vi "File - calendar tree.vi"(8 "error in (no error)":errorcluster) -> (0 "error out":errorcluster)   [LabVIEW 2026, in "Tests.lvlib"]
doc: "Integration test (Caraya). Verifies a statement logged through the Logger reaches a single registered appender. Launches a manager with the default file disabled and a queue-mode relay capture probe (Open Test Mgr), logs one INFO statement, dequeues from the capture queue with a timeout, and asserts it was delivered and its message matches. Tears down with Close Test Mgr regardless of assertion outcome (SRS-LMBR-019). Uses the manager fixture; no temp root needed.\n\nImplements LMBR-T-029 -> SRS-019. Assert-level IDs: Test-ID-Assert-Checklist.md."
uses:
  Tests.lvlib
  src/TypeDefs/Severity.ctl
  src/TypeDefs/FileAppenderConfig.ctl
  src/TypeDefs/AppenderConfig.ctl
  src/TypeDefs/Filter.ctl
  src/TypeDefs/FilterMode.ctl
  src/TypeDefs/DropPolicy.ctl
  src/TypeDefs/FileConfig.ctl
  <vilib>/addons/_JKI Toolkits/Caraya/classes/Assert/Assert False.vi
  <vilib>/addons/_JKI Toolkits/Caraya/classes/Assert/Assert True.vi
  <vilib>/addons/_JKI Toolkits/Caraya/classes/Test/Test.lvclass
  src/Lumberjack.lvlib
  src/Public/Logger.lvclass/Logger.lvclass
  <vilib>/addons/_JKI Toolkits/Caraya/classes/Assert/Assert.lvclass
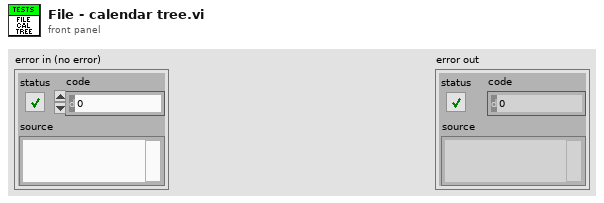
[diagram p1: front panel]
types:
  T1 = typedef "Lumberjack.lvlib/Severity.ctl" = enum16{"OFF", "FATAL", "ERROR", "WARN", "INFO", "DEBUG", "TRACE", "ALL"}
  T2 = typedef "Lumberjack.lvlib/FileAppenderConfig.ctl" = cluster{"common":T3, "file":T7}
  T3 = typedef "Lumberjack.lvlib/AppenderConfig.ctl" = cluster{"id":string, "threshold":T1, "filter":T4, "queueBound":i32, "dropPolicy":T6, "useUTC":bool}
  T4 = typedef "Lumberjack.lvlib/Filter.ctl" = cluster{"mode":T5, "levelMin":T1, "levelMax":T1, "tagPrefix":string}
  T5 = typedef "Lumberjack.lvlib/FilterMode.ctl" = enum16{"Mirror", "Routed"}
  T6 = typedef "Lumberjack.lvlib/DropPolicy.ctl" = enum16{"DropOldest", "DropNewest", "LevelAware"}
  T7 = typedef "Lumberjack.lvlib/FileConfig.ctl" = cluster{"rootFolder":path, "maxFileSize":i64, "maxFileCount":i32, "baseName":string, "extension":string, "delimiter":string, "calendarFolderTree":bool}
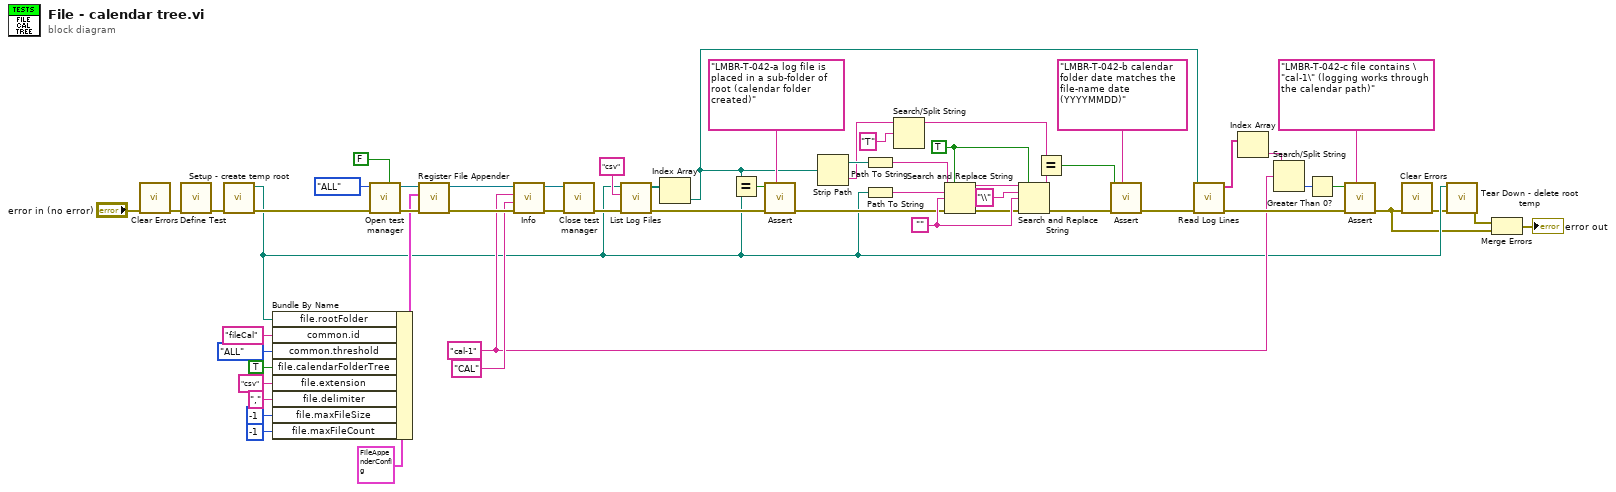
[diagram p0: block diagram]
diagram:
  w19 = TRUE ("replace all? (F)")
  w21 = ""
  w30 = "cal-1" ("message")
  n1 = call <vilib>:"Clear Errors.vi"("error in (no error)"="error in (no error)") -> ("error out"=w5:errorcluster)  [unwired: 5 in, 1 out]
  n2 = call <vilib>:"Define Test.vi"("error in (no error)"=w5) -> ("error out"=w57:errorcluster)  [unwired: 9 in, 1 out]
  n3 = call "Setup - create temp root.vi"("error in (no error)"=w57) -> ("error out"=w27:errorcluster, "tempRoot"=w8:path)  [unwired: 9 in]
  n4 = Bundle By Name(cluster=T2 {"common"={"id"="", "threshold"=enum."INFO", "filter"={"mode"=enum."Mirror", "levelMin"=enum."INFO", "levelMax"=enum."INFO", "tagPrefix"=""}, "queueBound"=0, "dropPolicy"=enum."DropOldest", "useUTC"=FALSE}, "file"={"rootFolder"=path "", "maxFileSize"=0, "maxFileCount"=0, "baseName"="", "extension"="", "delimiter"="", "calendarFolderTree"=FALSE}} ("FileAppenderConfig"), "file.rootFolder"=w8, "common.id"="fileCal", "common.threshold"=Severity."ALL", "file.calendarFolderTree"=TRUE, "file.extension"="csv", "file.delimiter"=",", "file.maxFileSize"=i64 -1, "file.maxFileCount"=-1) -> (w51:T2)
  n5 = call "Open test manager.vi"("enableDefaultFile"=FALSE, "error in (no error)"=w27, "globalThreshold"=Severity."ALL") -> ("error out"=w55:errorcluster, "Logger out"=w50:refnum<class "Logger.lvclass">)  [unwired: 7 in]
  n6 = call "Register File Appender.vi"("error in (no error)"=w55, "FileAppenderConfig"=w51, "Logger in"=w50) -> ("error out"=w54:errorcluster, "Logger out"=w49:refnum<class "Logger.lvclass">)  [unwired: 6 in, 1 out]
  n7 = call "Info.vi"("error in (no error)"=w54, "sourceTag"="CAL", "message"=w30, "Logger in"=w49) -> ("error out"=w46:errorcluster, "Logger out"=w45:refnum<class "Logger.lvclass">)  [unwired: 6 in]
  n8 = call "Close test manager.vi"("error in (no error)"=w46, "Logger in"=w45) -> ("error out"=w17:errorcluster)  [unwired: 7 in]
  n9 = call "List Log Files.vi"("error in (no error)"=w17, "extension"="csv", "rootFolder"=w8) -> ("error out"=w28:errorcluster, "filePaths"=w43:path[])  [unwired: 6 in, 1 out]
  n10 = Index Array(array=w43) -> (element=w7:path)  [unwired: 1 in]
  n11 = Equal?(x=w7, y=w8) -> (x = y?=w25:bool)
  n12 = call-poly <vilib>:"Assert.vi"("Label"="LMBR-T-042-a log file is placed in a sub-folder of root (calendar folder created)", "error in (no error)"=w28, "False?"=w25) -> ("error out"=w15:errorcluster)  [unwired: 7 in, 1 out]
  n13 = Strip Path(path=w7) -> (stripped path=w16:path, name=w14:string)
  n14 = Path To String(path=w16) -> (string=w24:string)
  n15 = Path To String(path=w8) -> (string=w23:string)
  n16 = Search/Split String(string=w14, search string/char (-)="T") -> (substring before match=w11:string)  [unwired: 1 in, 2 out]
  n17 = Search and Replace String(replace all?=w19, input string=w24, search string=w23, replace string=w21, error in=w15) -> (result string=w20:string, error out=w18:errorcluster)  [unwired: 3 in, 2 out]
  n18 = Search and Replace String(replace all?=w19, input string=w20, search string="\\", replace string=w21, error in=w18) -> (result string=w12:string, error out=w9:errorcluster)  [unwired: 3 in, 2 out]
  n19 = Equal?(x=w11, y=w12) -> (x = y?=w10:bool)
  n20 = call-poly <vilib>:"Assert.vi"("Label"="LMBR-T-042-b calendar folder date matches the file-name date (YYYYMMDD)", "error in (no error)"=w9, "True?"=w10) -> ("error out"=w40:errorcluster)  [unwired: 7 in, 1 out]
  n21 = call "Read Log Lines.vi"("error in (no error)"=w40, "filePath"=w7) -> ("error out"=w35:errorcluster, "lines"=w31:string[])  [unwired: 8 in]
  n22 = Index Array(array=w31) -> (element=w29:string)  [unwired: 1 in]
  n23 = Search/Split String(string=w29, search string/char (-)=w30) -> (offset of match=w42:i32)  [unwired: 1 in, 2 out]
  n24 = Greater Than 0?(x=w42) -> (x > 0?=w41:bool)
  n25 = call-poly <vilib>:"Assert.vi"("Label"="LMBR-T-042-c file contains \"cal-1\" (logging works through the calendar path)", "error in (no error)"=w35, "True?"=w41) -> ("error out"=w2:errorcluster)  [unwired: 7 in, 1 out]
  n26 = call <vilib>:"Clear Errors.vi"("error in (no error)"=w2) -> ("error out"=w1:errorcluster)  [unwired: 5 in, 1 out]
  n27 = call "Tear Down - delete root temp.vi"("error in (no error)"=w1, "tempRoot"=w8) -> ("error out"=w4:errorcluster)  [unwired: 9 in]
  n28 = Merge Errors(w4, w2) -> (→"error out":errorcluster)
